vi "Link Status.vi"(8 "Error In":errorcluster, 9 "Remote Path":string, 10 "Attributes In":refnum<class "SFTP Attributes.lvclass">, 11 "SFTP In":refnum<class "SFTP.lvclass">) -> (0 "Error Out":errorcluster, 2 "Attributes Out":refnum<class "SFTP Attributes.lvclass">, 3 "SFTP Out":refnum<class "SFTP.lvclass">)   [LabVIEW 2018, in "Toolkit.lvlib" / "SFTP.lvclass"]
uses:
  SFTP.lvclass
  SFTP Attributes/SFTP Attributes.lvclass
  SFTP.lvclass/SFTP.ctl
  SFTP Attributes/SFTP Attributes.lvclass/SFTP Attributes.ctl
  Session/Session.lvclass/Session.ctl
  SSH/SSH.lvclass/SSH.ctl
  Toolkit.lvlib
  Session/Session.lvclass
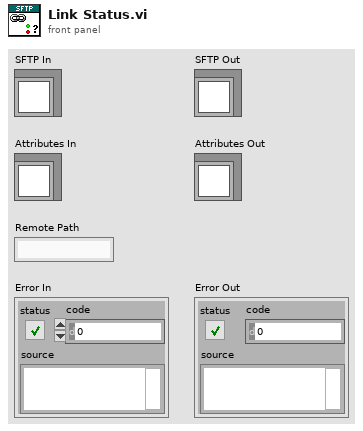
[diagram p1: front panel]
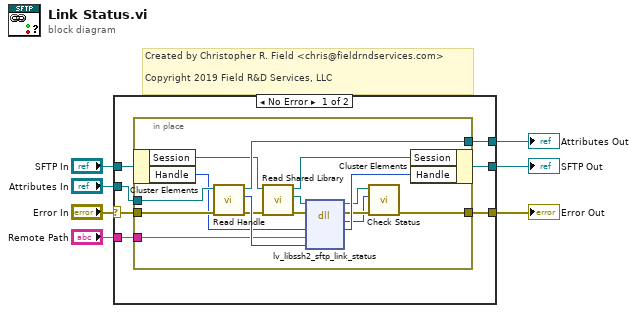
[diagram p0: block diagram]
diagram:
  # "Created by Christopher R. Field <chris@fieldrndservices.com>\n\nCopyright 2019 Field R&D Services, LLC"
  n1 = case shown="No Error" "Error In" {
    selector: "Error In" -> [w14 w33]
    tunnel: [w13 w33] -> w6
    tunnel: "Attributes In" -> [w12 w32]
    tunnel: [w11 w32] -> w4
    tunnel: "SFTP In" -> [w10 w31]
    tunnel: [w9 w31] -> w2
    tunnel: "Remote Path" -> [w8 _]
    frame No Error {
      n2 = in-place {
        in-place-border: w14 -> [w23]
        in-place-border: [w26] -> w13
        in-place-border: w12 -> [w25]
        in-place-border: [w22] -> w11
        in-place-border: w8 -> [w15]
        n3 = in-place-cluster #1(w10) -> ("Session"=w21:refnum<class "Session.lvclass">, "Handle"=w16:u64)
        n4 = call "Read Handle.vi"("Error In"=w23, "SFTP Attributes In"=w25) -> ("Error Out"=w19:errorcluster, "Handle"=w24:u64, "SFTP Attributes Out"=w22:refnum<class "SFTP Attributes.lvclass">)  [unwired: 7 in]
        n5 = call "Read Shared Library.vi"("Error In"=w19, "Session In"=w21) -> ("Erorr Out"=w18:errorcluster, "libssh2lv Shared Library"=w17:path, "Session Out"=w20:refnum<class "Session.lvclass">)  [unwired: 7 in]
        n6 = dll-call lib="libssh2lv.*" fn="lv_libssh2_sftp_link_status"(path in=w17, error in=w18, "handle"=w16, "path"=w15, "attributes"=w24) -> (path out=w28:path, error out=w29:errorcluster, "status"=w27:i32, "handle"=w30:u64)  [unwired: 3 in]
        n7 = call "Check Status.vi"("Error In"=w29, "Status"=w27, "lv-libssh2 Shared Library In"=w28) -> ("Error Out"=w26:errorcluster)  [unwired: 7 in, 1 out]
        n8 = in-place-cluster #1("Session"=w20, "Handle"=w30) -> (w9:refnum<class "SFTP.lvclass">)
      }
    }
    frame Error {
    }
  }
  "Error Out" <- w6
  "Attributes Out" <- w4
  "SFTP Out" <- w2
